vi "Pixel count.vi"(1 "Input":dbl[](array[numeric]), 2 "shift":i8) -> (0 "Output":dbl[](array[numeric]))   [LabVIEW 2012]
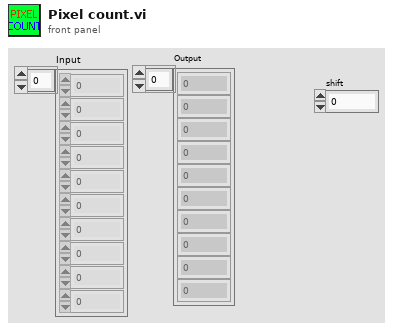
[diagram p1: front panel]
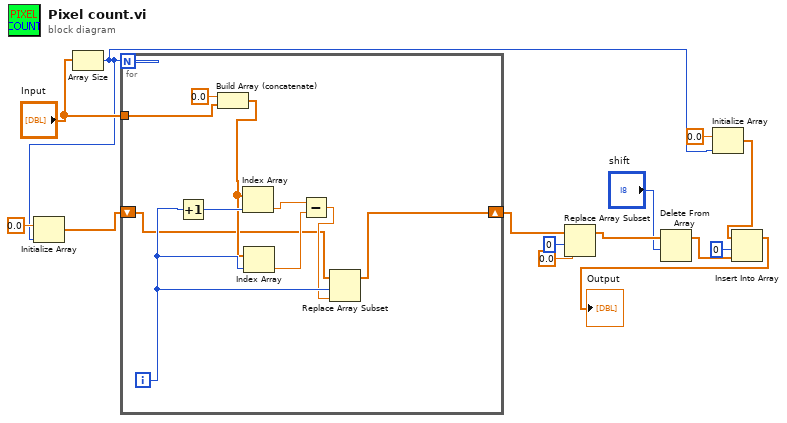
[diagram p0: block diagram]
diagram:
  n1 = Array Size(array="Input") -> (size(s)=w5:i32)
  n2 = Initialize Array(0.0 ("element"), w5) -> (w12:dbl[])
  n3 = for {
    N: w5 -> [_]
    tunnel: "Input" -> [w23]
    shift-right: [w16] -> w11
    shift-left: w12 -> [w15]
    i -> [w21]
    n4 = Increment(x=w21) -> (x+1=w22:i32)
    n5 = Build Array (concatenate)(0.0 ("element"), w23) -> (w20:dbl[])
    n6 = Index Array(array=w20, index=w22) -> (element=w19:dbl)
    n7 = Index Array(array=w20, index=w21) -> (element=w18:dbl)
    n8 = Subtract(x=w19, y=w18) -> (x-y=w17:dbl)
    n9 = Replace Array Subset(array=w15, new element=w17, index=w21) -> (w16:dbl[])
  }
  n10 = Replace Array Subset(array=w11, new element=0.0 ("new element/subarray"), index=0) -> (w8:dbl[])
  n11 = Delete From Array(array=w8, length="shift") -> (array with subset deleted=w3:dbl[])  [unwired: 1 in, 1 out]
  n12 = Initialize Array(0.0 ("element"), w5) -> (w4:dbl[])
  n13 = Insert Into Array(array=w4, index=0, new element=w3) -> (→"Output":dbl[])
